vi "PV OnTool Miscellaneous.vi"(8 "error in (no error)":errorcluster, 9 "PV OnTool Miscellaneous - Cluster":T1={"Parameter"=0, "Parameter\nread only<->describe"=FALSE, "Unit adress"=1, "Configuration output K1"=0, "Remote operations mode"=0, "Characteristic analog input "=0} {"Characteristic analog input" items=[" proportional rotation speed", " proportional rotation speed  <=15%", " proportional rotation speed >= 80%"]; "Remote operations mode" items=[" operations via remote", " operations via PV-Protocol"]; "Configuration output K1" items=[" User controlled", " Drive synchron", " Drive invers synchron"]; "Unit adress" min=1 max=255 step=1; "Parameter" items=[" Configuration output K1", " Remote operations mode", " Characteristic analog input", " Actual error code (read only)", " Software version electronic drive unit  (read only)", " Interlock ok  (read only)", " Unit type electronic drive unit", " Software version controller (read only)", " Hardware version (read only)", " Unit address", " Error acknowledgement"]}, 10 "Adress of unit":u16=1 max=999 step=1, 11 "VISA session":refnum<visa-resource-name>) -> (0 "error out":errorcluster, 2 "response (data)":string, 3 "dup VISA session":refnum<visa-resource-name>)   [LabVIEW 2016, in "Pfeiffer Vacuum.lvlib"]
doc: "There are 11 parameters available, only one of which can be enabled at a time. \n\n0 - Configuration output K1 (default) (Para. 024)\n1 - Remote operations mode (Para. 028)\n2 - Characteristic analog input (Para. 033)\n3 - Actual error code (read only) (Para. 303)\n4 - Software version process unit (read only) (Para.312)\n5 - Interlock ok (read only) (Para. 345)\n6 - Unit type electronic drive unit (Para. 349)\n7 - Software version controller (read only) (Para. 352)\n8 - Hardware version (read only) (Para. 354)\n9 - Unit address (Para. 797)\n10 - Error acknowledgement (Para. 009)\n\nNote: The 4 controls right of this one will set the appropriate values for the selected parameter. Any settings for an parameter that is not selected will be ignored. If a value is out of range, it will be changed to either the upper or the lower limit of the range."
uses:
  Pfeiffer Vacuum.lvlib
  PV OnTool Miscelaneous - Cluster.ctl
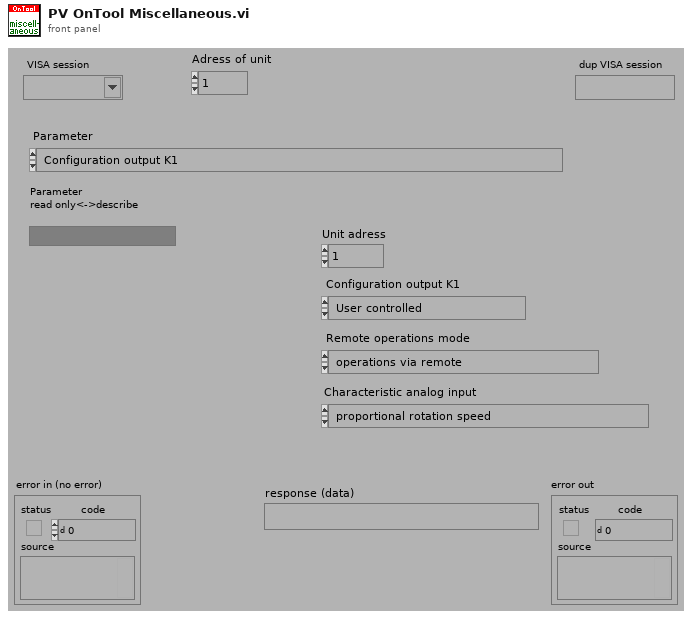
[diagram p1: front panel]
types:
  T1 = typedef "Pfeiffer Vacuum.lvlib/PV OnTool Miscelaneous - Cluster.ctl" = cluster{"Parameter":u16, "Parameter\nread only<->describe":bool, "Unit adress":i16, "Configuration output K1":u16, "Remote operations mode":u16, "Characteristic analog input ":u16}
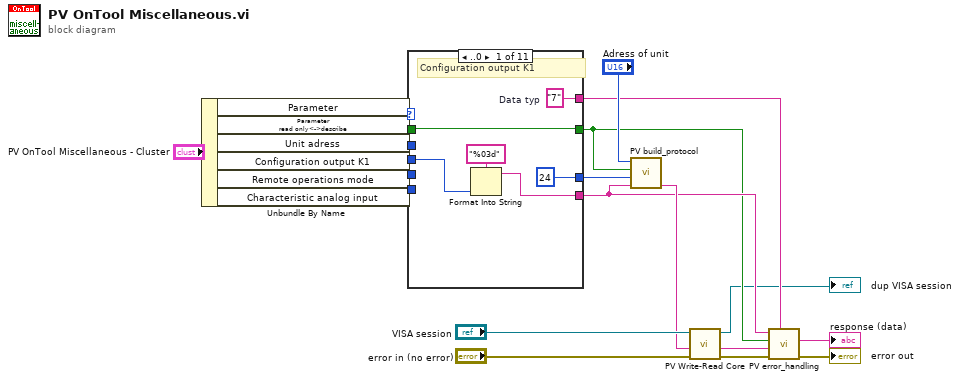
[diagram p0: block diagram]
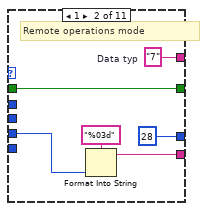
[diagram p2: hidden frame]
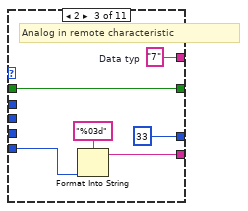
[diagram p3: hidden frame]
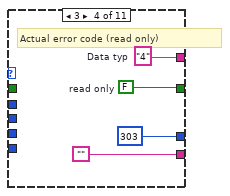
[diagram p4: hidden frame]
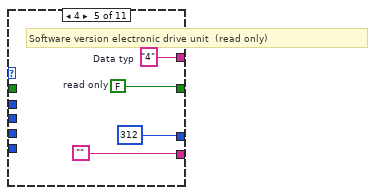
[diagram p5: hidden frame]
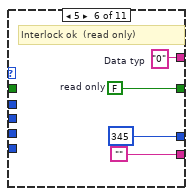
[diagram p6: hidden frame]
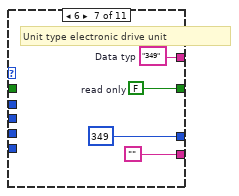
[diagram p7: hidden frame]
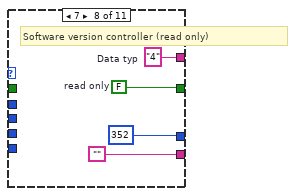
[diagram p8: hidden frame]
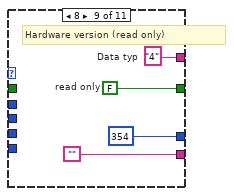
[diagram p9: hidden frame]
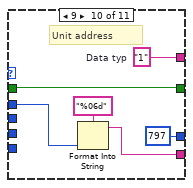
[diagram p10: hidden frame]
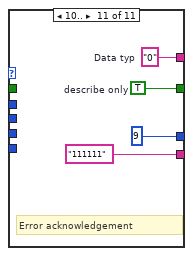
[diagram p11: hidden frame]
diagram:
  n1 = Unbundle By Name("PV OnTool Miscellaneous - Cluster") -> ("Parameter"=w17:u16, "Parameter\nread only<->describe"=w16:bool, "Unit adress"=w15:i16, "Configuration output K1"=w14:u16, "Remote operations mode"=w13:u16, "Characteristic analog input"=w12:u16)
  n2 = case shown="..0" w17 {
    tunnel: [u16 24 ("Parameter-number") u16 28 ("Parameter-number") u16 33 ("Parameter-number") u16 303 ("Parameter-number") u16 312 ("Parameter-number") u16 345 ("Parameter-number") u16 349 ("Parameter-number") u16 352 ("Parameter-number") u16 354 ("Parameter-number") u16 797 ("Parameter-number") u16 9 ("Parameter-number")] -> w19
    tunnel: [w23 w29 w35 "" "" "" "" "" "" w68 "111111" ("Data")] -> w5
    tunnel: [w25 w31 w37 w41 w45 w50 w54 w58 w62 w65 w72] -> w4
    tunnel: w16 -> [w25 w31 w37 _ _ _ _ _ _ w65 _]
    tunnel: w15 -> [_ _ _ _ _ _ _ _ _ w64 _]
    tunnel: w14 -> [w22 _ _ _ _ _ _ _ _ _ _]
    tunnel: w13 -> [_ w28 _ _ _ _ _ _ _ _ _]
    tunnel: w12 -> [_ _ w34 _ _ _ _ _ _ _ _]
    tunnel: [w21 w27 w33 w39 w43 w47 w51 w55 w59 w63 w69] -> w6
    frame ..0 {
      w21 = "7"  # Data typ
      # "Configuration output K1"
      n3 = Format Into String(format string="%03d" ("Format-String"), w22) -> (resulting string=w23:string)  [unwired: 2 in, 1 out]
    }
    frame 1 {
      w27 = "7"  # Data typ
      # "Remote operations mode"
      n4 = Format Into String(format string="%03d" ("Format-String"), w28) -> (resulting string=w29:string)  [unwired: 2 in, 1 out]
    }
    frame 2 {
      w33 = "7"  # Data typ
      # "Analog in remote characteristic"
      n5 = Format Into String(format string="%03d" ("Format-String"), w34) -> (resulting string=w35:string)  [unwired: 2 in, 1 out]
    }
    frame 3 {
      w39 = "4"  # Data typ
      w41 = FALSE  # read only
      # "Actual error code (read only)"
    }
    frame 4 {
      w43 = "4"  # Data typ
      w45 = FALSE  # read only
      # "Software version electronic drive unit  (read only)"
    }
    frame 5 {
      w47 = "0"  # Data typ
      w50 = FALSE  # read only
      # "Interlock ok  (read only)"
    }
    frame 6 {
      w51 = "349"  # Data typ
      w54 = FALSE  # read only
      # "Unit type electronic drive unit"
    }
    frame 7 {
      w55 = "4"  # Data typ
      w58 = FALSE  # read only
      # "Software version controller (read only)"
    }
    frame 8 {
      w59 = "4"  # Data typ
      w62 = FALSE  # read only
      # "Hardware version (read only)"
    }
    frame 9 {
      w63 = "1"  # Data typ
      # "Unit address"
      n6 = Format Into String(format string="%06d" ("Format-String"), w64) -> (resulting string=w68:string)  [unwired: 2 in, 1 out]
    }
    frame 10.. {
      w69 = "0"  # Data typ
      w72 = TRUE  # describe only
      # "Error acknowledgement"
    }
  }
  n7 = call "PV build_protocol.vi"("Data"=w5, "Parameter-number"=w19, "parameter\nread<->describe"=w4, "Adress"="Adress of unit") -> ("output"=w9:string)  [unwired: 3 in]
  n8 = call "PV Write-Read Core.vi"("error in"="error in (no error)", "Write data in"=w9, "VISA session"="VISA session") -> ("error out"=w7:errorcluster, "response (data) out"=w8:string, "dup VISA session"=→"dup VISA session":refnum<visa-resource-name>)  [unwired: 2 in]
  n9 = call "PV error_handling.vi"("Data Typ in"=w6, "error in"=w7, "response (data) in"=w8, "Parameter\nread only<->describe"=w4, "data in"=w5) -> ("error out"=→"error out":errorcluster, "Data out"=→"response (data)":string)  [unwired: 4 in, 1 out]
